vi "Sort Hands.vi"(11 "Array":refnum<class "Hand.lvclass">[](array[class])) -> (3 "Sorted":refnum<class "Hand.lvclass">[](array[class]))   [LabVIEW 2020]
uses:
  Hand/Hand.lvclass
  c4cfd050-3f65-41ae-917f-2c266e8d5b1d.vi
  c4cfd050-3f65-41ae-917f-2c266e8d5b1d.vi/0ef24ca0-c7f0-4e73-81b6-d4fe6aada9a9.vi
  c4cfd050-3f65-41ae-917f-2c266e8d5b1d.vi/0ef24ca0-c7f0-4e73-81b6-d4fe6aada9a9.vi/19e2e4cb-e3bb-4239-bd5f-680916605f5d.vi
  c4cfd050-3f65-41ae-917f-2c266e8d5b1d.vi/0ef24ca0-c7f0-4e73-81b6-d4fe6aada9a9.vi/f72612c1-738a-48a1-9fcf-3db66cb27fb3.vi
  c4cfd050-3f65-41ae-917f-2c266e8d5b1d.vi/0ef24ca0-c7f0-4e73-81b6-d4fe6aada9a9.vi/45406051-8994-464b-8b47-ac12a8cbadfa.vi
  c4cfd050-3f65-41ae-917f-2c266e8d5b1d.vi/0ef24ca0-c7f0-4e73-81b6-d4fe6aada9a9.vi/dd886480-778c-48b1-8e4a-d6890e1a60dd.vi
  c4cfd050-3f65-41ae-917f-2c266e8d5b1d.vi/0ef24ca0-c7f0-4e73-81b6-d4fe6aada9a9.vi/2e6e140f-e361-4312-a09e-e37273ac7fd1.vi
  c4cfd050-3f65-41ae-917f-2c266e8d5b1d.vi/0ef24ca0-c7f0-4e73-81b6-d4fe6aada9a9.vi/3589548e-4c68-4568-af05-72ab28470577.vi
  c4cfd050-3f65-41ae-917f-2c266e8d5b1d.vi/0ef24ca0-c7f0-4e73-81b6-d4fe6aada9a9.vi/cf64d4f5-91bd-4749-9577-68c6ded0155b.vi
  c4cfd050-3f65-41ae-917f-2c266e8d5b1d.vi/0ef24ca0-c7f0-4e73-81b6-d4fe6aada9a9.vi/6f6fefe9-f25b-4595-b26f-75715299a794.vi
  c4cfd050-3f65-41ae-917f-2c266e8d5b1d.vi/0ef24ca0-c7f0-4e73-81b6-d4fe6aada9a9.vi/c74ffb76-1048-4639-9a95-b6de96ba7014.vi
  Hand/Less Than.vi
  <vilib>/Comparison/Less/Less Functor/Less Functor.lvclass
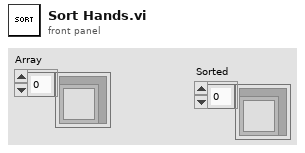
[diagram p1: front panel]
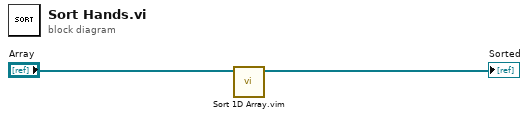
[diagram p0: block diagram]
diagram:
  n1 = call "Sort 1D Array.vim"("unsorted array"="Array") -> ("sorted array"=→"Sorted":refnum<class "Hand.lvclass">[])  [unwired: 10 in]
